vi "Set Load.vi"(8 "error in (no error)":errorcluster, 10 "Boolean":bool, 11 "Numeric":u16) -> (0 "error out":errorcluster)   [LabVIEW 2017]
uses:
  <vilib>/Platform/TimedLoop/XDataNode/timing_clust.ctl
  <vilib>/Platform/TimedLoop/XDataNode/nitl_modes.ctl
  <vilib>/Platform/TimedLoop/XDataNode/wakeup.ctl
  <vilib>/DAQmx/write.llb/DAQmx Write (Digital Bool 1Line 1Point).vi
  <vilib>/DAQmx/write.llb/DAQmx Write (Digital 1D Bool NChan 1Samp 1Line).vi
  <vilib>/DAQmx/miscellaneous.llb/DAQmx Fill In Error Info.vi
  <vilib>/Platform/TimedLoop/XDataNode/XDataNode.xnode
  <vilib>/Platform/TimedLoop/XDataNode/XDNodeRunTimeDep.lvlib
panel:
  in  "Period":i64=50
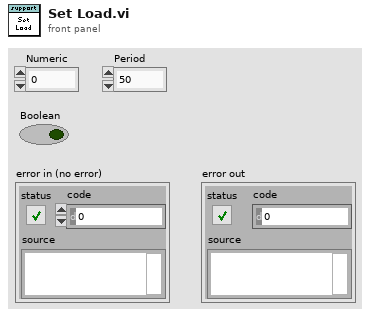
[diagram p1: front panel]
types:
  T1 = typedef "XDNodeRunTimeDep.lvlib/timing_clust.ctl" = cluster{"Expected End [f-1]":u64, "Actual End [f-1]":u64, "Finished Late? [f-1]":bool, "Expected End [i-1]":u64, "Actual End [i-1]":u64, "Finished Late? [i-1]":bool, "Expected Start [i]":u64, "Actual Start [i]":u64, "Expected Start [f]":u64, "Actual Start [f]":u64, "Source Name":string, "Structure Name":string, "Period":i64, "Deadline":i64, "Offset":i64, "Start":i64, "Priority":i32, "Timeout":i32, "Mode":T2, "Wakeup Reason":T3, "Error":errorcluster, "Source Type":string, "Secondary Source Type":string, "Global End Time":u64, "Global Start Time":u64, "Frame Duration":u64, "Iteration Duration":u64, "Assigned CPU":i32, "I/O Scan Engine Mode":u32}
  T2 = typedef "XDNodeRunTimeDep.lvlib/nitl_modes.ctl" = enum32{"No Change", "Process missed periods, maintain original phase", "Discard missed periods, maintain original phase", "Process missed periods, ignore original phase", "Discard missed periods, ignore original phase"}
  T3 = typedef "XDNodeRunTimeDep.lvlib/wakeup.ctl" = enum32{"Normal", "Aborted", "Asynchronous wakeup", "Timing source error", "Timed loop error", "Timeout"}
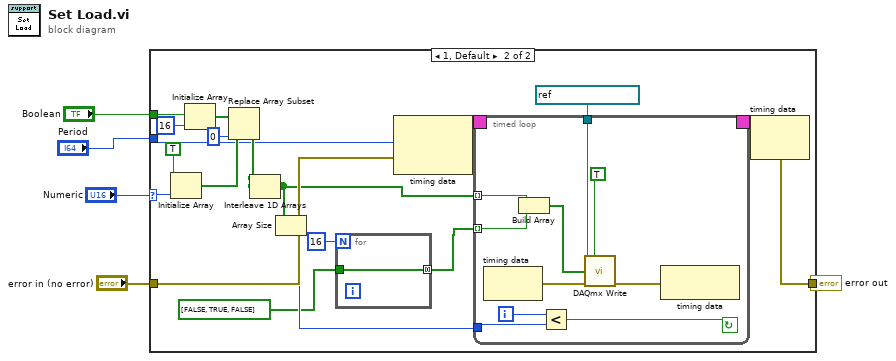
[diagram p0: block diagram]
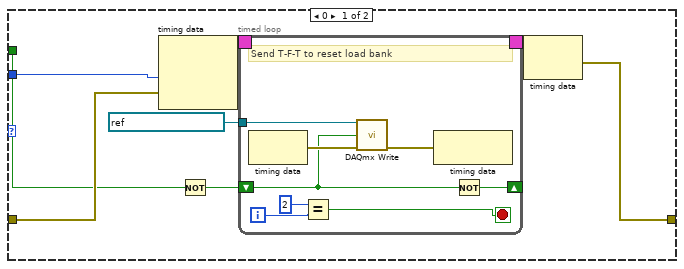
[diagram p2: hidden frame]
diagram:
  n1 = case shown="1, Default" "Numeric" {
    selector: "Numeric" -> [_ w43]
    tunnel: "error in (no error)" -> [w9 w47]
    tunnel: "Boolean" -> [w8 w41]
    tunnel: [w7 w48] -> w5
    tunnel: "Period" -> [w6 w33]
    frame 0 {
      n2 = node-c288(w6, w9) -> (w13:T1)  [unwired: 1 in]
      n3 = Not(x=w8) -> (.not. x?=w10:bool)
      n4 = timed-loop {
        timing: w13 -> [_]
        timing-out: [_] -> w12
        tunnel: refnum<k21> "PrecorLoadReset" -> [w21]
        shift-right: [w14] -> _
        shift-left: w10 -> [w15]
        i -> [w18]
        stop <- w16 stop-if-true
        # "Send T-F-T to reset load bank"
        n5 = node-c288() -> (w20:errorcluster)  [unwired: 1 in]
        n6 = Equal?(x=2, y=w18) -> (x = y?=w16:bool)
        n7 = call-poly <vilib>:"DAQmx Write.vi"("task/channels in"=w21, "data"=w15, "error in"=w20) -> ("error out"=w19:errorcluster)  [unwired: 10 in, 2 out]
        n8 = node-c288(w19) -> ()  [unwired: 1 out]
        n9 = Not(x=w15) -> (.not. x?=w14:bool)
      }
      n10 = node-c288(w12) -> (w7:errorcluster)
    }
    frame 1, Default {
      n11 = Initialize Array(TRUE, w43) -> (w38:bool[])
      n12 = Initialize Array(w41, 16 ("dimension size")) -> (w39:bool[])
      n13 = Replace Array Subset(array=w39, new element=w38, index=0) -> (w36:bool[])
      n14 = Interleave 1D Arrays(w36, w36, w36) -> (w34:bool[])
      n15 = Array Size(array=w34) -> (size(s)=w46:i32)
      n16 = for {
        N: 16 -> [_]
        tunnel: bool[] [FALSE, TRUE, FALSE] -> [w52]
        tunnel: [w52] -> w35 mode=concatenating
      }
      n17 = node-c288(w33, w47) -> (w50:T1)
      n18 = timed-loop {
        timing: w50 -> [_]
        timing-out: [_] -> w49
        tunnel: refnum<k21> "PrecorLoadSet" -> [w62]
        tunnel: w34 -> [w55] mode=indexing
        tunnel: w46 -> [w57]
        tunnel: w35 -> [w53] mode=indexing
        i -> [w58]
        stop <- w56 continue-if-true
        n19 = node-c288() -> (w61:errorcluster)  [unwired: 1 in]
        n20 = Build Array(w55, w53) -> (w54:bool[])
        n21 = Less?(x=w58, y=w57) -> (x < y?=w56:bool)
        n22 = call-poly <vilib>:"DAQmx Write.vi"("task/channels in"=w62, "auto start"=TRUE, "data"=w54, "error in"=w61) -> ("error out"=w60:errorcluster)  [unwired: 9 in, 2 out]
        n23 = node-c288(w60) -> ()  [unwired: 1 out]
      }
      n24 = node-c288(w49) -> (w48:errorcluster)
    }
  }
  "error out" <- w5
